vi "HV_ReadHV.vi"(8 "Run":i32, 11 "PMT":string[](array[string])) -> (0 "Voltages":string[](array[string]), 3 "PMT Out":string[](array[string]))   [LabVIEW 2019]
panel:
  out "array w/ subset deleted":dbl[][](array[numeric])
  out "appended path":path
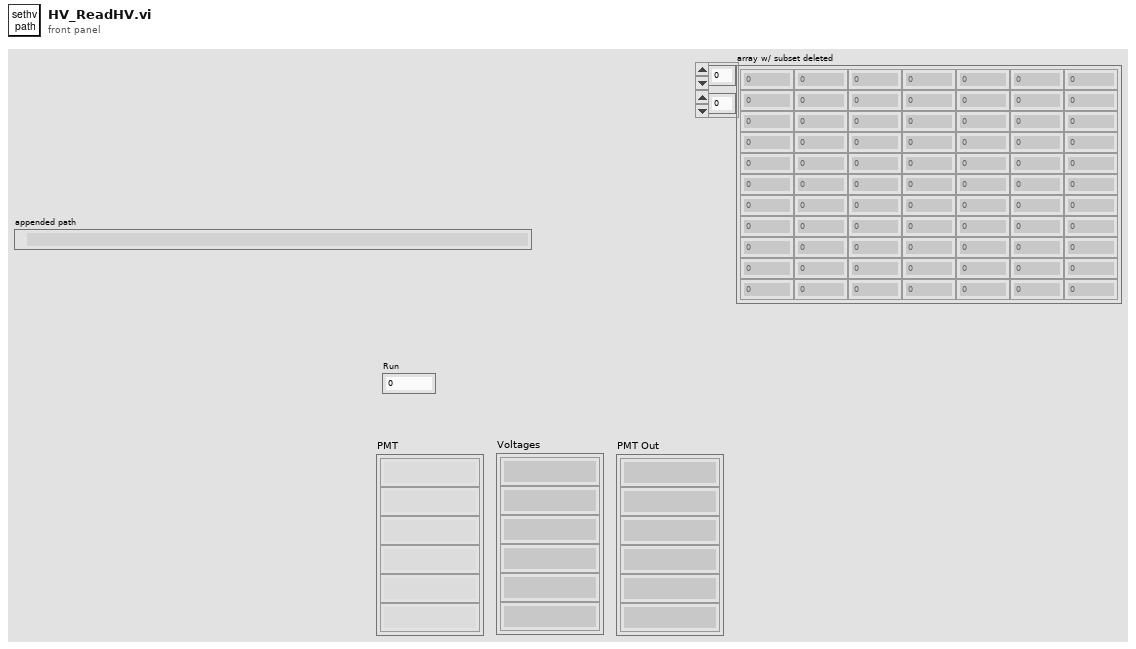
[diagram p1: front panel]
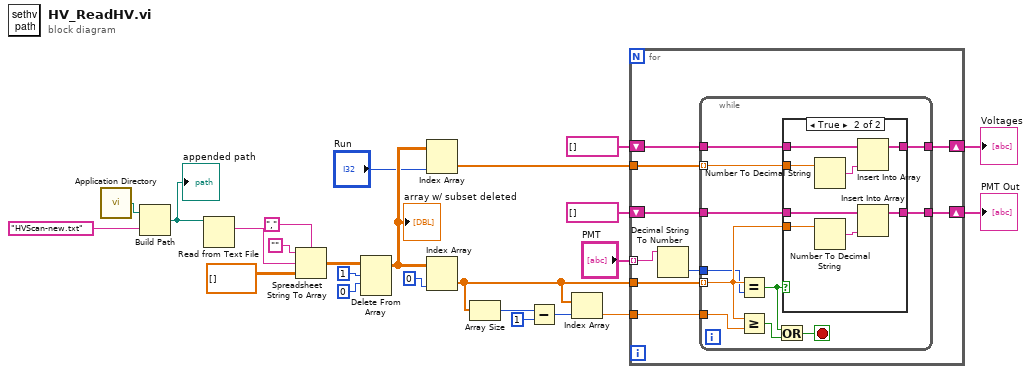
[diagram p0: block diagram]
diagram:
  n1 = call <vilib>:"Application Directory.vi"() -> ("Application Directory"=w23:path)
  n2 = Build Path(base path=w23, name or relative path="HVScan-new.txt") -> (appended path=w22:path)
  "appended path" <- w22
  n3 = Read from Text File(file (use dialog)=w22) -> (text=w21:string)  [unwired: 3 in, 3 out]
  n4 = Spreadsheet String To Array(delimiter (Tab)=",", format string="", spreadsheet string=w21, array type (2D Dbl)=dbl[][] []) -> (array=w17:dbl[][])
  n5 = Delete From Array(array=w17, length=1, index (row)=0) -> (array with subset deleted=w7:dbl[][])  [unwired: 1 in, 1 out]
  "array w/ subset deleted" <- w7
  n6 = Index Array(array=w7, index (col)="Run") -> (element=w6:dbl[])  [unwired: 1 in]
  n7 = Index Array(array=w7, index (col)=0 ("index (row)")) -> (element=w12:dbl[])  [unwired: 1 in]
  n8 = Array Size(array=w12) -> (size(s)=w11:i32)
  n9 = Subtract(x=w11, y=1) -> (x-y=w9:i32)
  n10 = Index Array(array=w12, index=w9) -> (element=w8:dbl)
  n11 = for {
    tunnel: w12 -> [w33]
    tunnel: "PMT" -> [w32] mode=indexing
    tunnel: w8 -> [w30]
    tunnel: w6 -> [w29]
    shift-right: [w27] -> w4
    shift-left: string[] [] -> [w28]
    shift-right: [w26] -> w3
    shift-left: string[] [] -> [w25]
    n12 = Decimal String To Number(string=w32) -> (number=w31:i32)  [unwired: 2 in, 1 out]
    n13 = while {
      tunnel: w33 -> [w41] mode=indexing
      tunnel: w31 -> [w40]
      tunnel: w30 -> [w39]
      tunnel: w29 -> [w38] mode=indexing
      tunnel: w28 -> [w37]
      tunnel: [w36] -> w27
      tunnel: [w35] -> w26
      tunnel: w25 -> [w34]
      stop <- w44 stop-if-true
      n14 = Equal?(x=w41, y=w40) -> (x = y?=w42:bool)
      n15 = Greater Or Equal?(x=w41, y=w39) -> (x >= y?=w43:bool)
      n16 = Or(x=w42, y=w43) -> (x .or. y?=w44:bool)
      n17 = case shown="True" w42 {
        tunnel: w41 -> [_ w54]
        tunnel: w38 -> [_ w50]
        tunnel: w37 -> [w46 w53]
        tunnel: [w46 w52] -> w36
        tunnel: [w45 w49] -> w35
        tunnel: w34 -> [w45 w48]
        frame False {
        }
        frame True {
          n18 = Number To Decimal String(number=w50) -> (decimal integer string=w51:string)  [unwired: 1 in]
          n19 = Number To Decimal String(number=w54) -> (decimal integer string=w47:string)  [unwired: 1 in]
          n20 = Insert Into Array(array=w53, new element=w51) -> (w52:string[])  [unwired: 1 in]
          n21 = Insert Into Array(array=w48, new element=w47) -> (w49:string[])  [unwired: 1 in]
        }
      }
    }
  }
  "Voltages" <- w4
  "PMT Out" <- w3
